vi "ActorDatabase-PerformQuery.vi"(8 "error in (no error)":errorcluster, 11 "Database-Actor in":refnum<class "Database-Actor.lvclass">) -> (0 "error out":errorcluster, 2 "Payload To Actor":string, 3 "Database-Actor out":refnum<class "Database-Actor.lvclass">)   [LabVIEW 2013, in "Database-Actor.lvclass"]
uses:
  Database-Actor.lvclass
  Database-Actor.lvclass/Database-Actor.ctl
  ftw-dataflow/Actor/src/Utility/FTW-Actor-Configuration.ctl
  ftw-dataflow/Core/src/JSON/FTW-JSON-RegexParse.vi
  ftw-dataflow/Core/src/Error/FTW-ERR-ThrowGenericError.vi
  ftw-dataflow/Core/src/Container/FTW-Container-Construct.vi
  ftw-dataflow/Core/src/Container/FTW-Container-Load-JSON.vi
  ftw-dataflow/Core/src/Container/FTW-Container-Destroy.vi
  ftw-dataflow/Core/utils/CodeGen/JSON Deserialize/FTW-JSON-Deserialize.xnode
  ftw-dataflow/Actor/src/FTW-Actor.lvlib
  Reuse Library/Database API/Database-API.lvclass
  ftw-dataflow/Core/src/Container/FTW-Container.lvclass
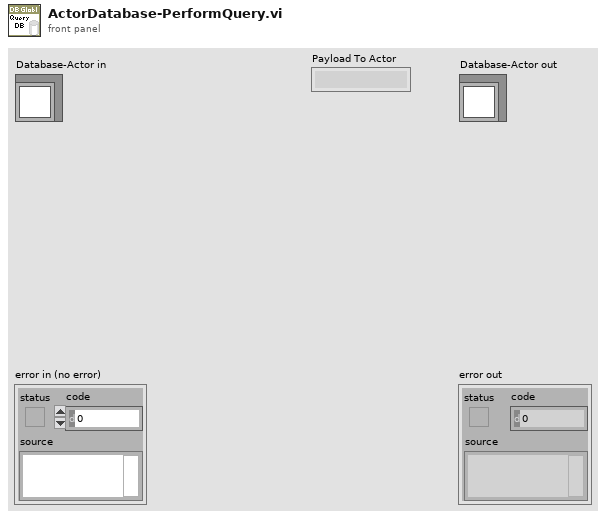
[diagram p1: front panel]
types:
  T1 = typedef "FTW-Actor.lvlib/FTW-Actor-Configuration.ctl" = string
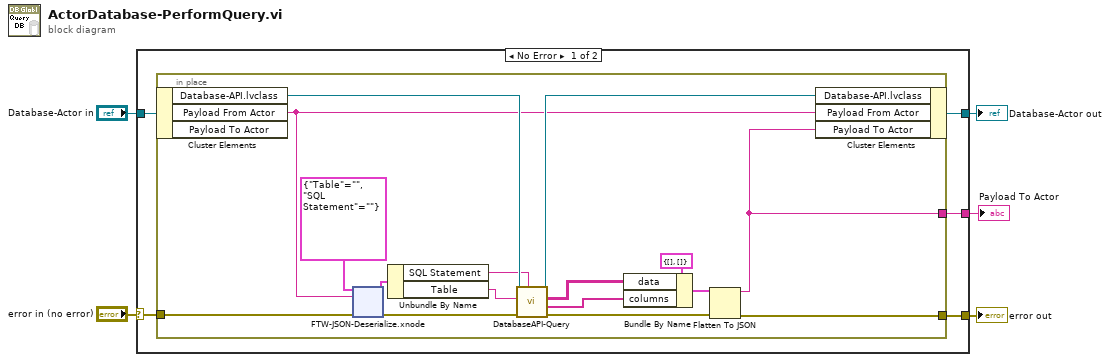
[diagram p0: block diagram]
diagram:
  n1 = case shown="No Error" "error in (no error)" {
    selector: "error in (no error)" -> [w10 w61]
    tunnel: [w9 w61] -> w4
    tunnel: [w7 w60] -> w2
    tunnel: "Database-Actor in" -> [w8 w60]
    tunnel: [w6 _] -> w1
    frame No Error {
      n2 = in-place {
        in-place-border: w10 -> [w14]
        in-place-border: [w13] -> w9
        in-place-border: [w12] -> w6
        n3 = in-place-cluster #1(w8) -> ("Database-API.lvclass"=w25:refnum<class "Database-API.lvclass">, "Payload From Actor"=w19:string)  [unwired: 1 out]
        n4 = xnode "FTW-JSON-Deserialize.xnode"("Data Type and Default Values"=cluster{"Table":T1, "SQL Statement":T1} {"Table"="", "SQL Statement"=""}, "JSON String"=w19, "error in"=w14) -> ("Populated Values"=w23:cluster{"Table":T1, "SQL Statement":T1}, "error out"=w24:errorcluster)
        n5 = Unbundle By Name(w23) -> ("SQL Statement"=w21:T1, "Table"=w22:T1)
        n6 = call "DatabaseAPI-Query.vi"("optional clause"=w21, "error in (no error)"=w24, "Table"=w22, "Database-API in"=w25) -> ("error out"=w15:errorcluster, "columns"=w11:string[], "data"=w16:string[][], "Database-API out"=w20:refnum<class "Database-API.lvclass">)  [unwired: 4 in]
        n7 = Bundle By Name(cluster=cluster{"data":string[][], "columns":string[]} {"data"=[], "columns"=[]}, "data"=w16, "columns"=w11) -> (w17:cluster{"data":string[][], "columns":string[]})
        n8 = Flatten To JSON(anything=w17, error in (no error)=w15) -> (JSON string=w12:string, 11:w13:errorcluster)  [unwired: 1 in]
        n9 = in-place-cluster #1("Database-API.lvclass"=w20, "Payload From Actor"=w19, "Payload To Actor"=w12) -> (w7:refnum<class "Database-Actor.lvclass">)
      }
    }
    frame Error {
    }
  }
  "error out" <- w4
  "Database-Actor out" <- w2
  "Payload To Actor" <- w1
